vi "DrawFilledPolyOnImageGreyscale.vi"(4 "Thickness (Default: 1)":i32=1, 6 "Colour":u8=255, 7 "OpenCV Line Type (Default LINE_8)":T3=enum."LINE_8", 8 "error in (no error)":errorcluster, 9 "Point Type (Default: Any)":T1, 10 "Points":T2[](array[typedef]), 11 "Greyscale Image":refnum<data-value>) -> (0 "error out":errorcluster, 3 "Greyscale Image (Duplicate)":refnum<data-value>)   [LabVIEW 2020, in "g_ar_toolkit.image.lvlib"]
uses:
  g_ar_toolkit.image.lvlib
  Fill-Poly Points Type.ctl
  e24a04ad-8575-4d64-b8af-da4c51ecb9cd.vi
  Line Type.ctl
  g_ar_toolkit.common/Image Point (Integer).ctl
  g_ar_toolkit.common/g_ar_toolkit.common.lvlib
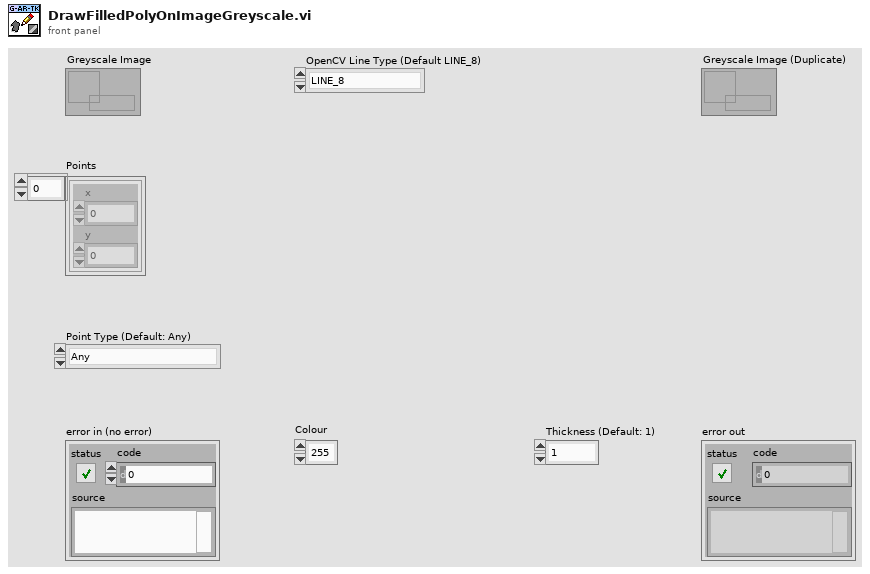
[diagram p1: front panel]
types:
  T1 = typedef "g_ar_toolkit.image.lvlib/Fill-Poly Points Type.ctl" = enum16{"Any", "Convex Only"}
  T2 = typedef "g_ar_toolkit.common.lvlib/Image Point (Integer).ctl" = cluster{"x":i32, "y":i32}
  T3 = typedef "g_ar_toolkit.image.lvlib/Line Type.ctl" = enum8{"FILLED", "LINE_4", "LINE_8", "LINE_AA"}
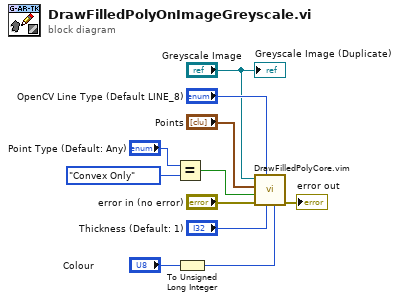
[diagram p0: block diagram]
diagram:
  n1 = Equal?(x="Point Type (Default: Any)", y=Fill-Poly_Points_Type."Convex Only") -> (x = y?=w2:bool)
  n2 = To Unsigned Long Integer(number="Colour") -> (unsigned 32bit integer=w6:u32)
  n3 = call "DrawFilledPolyCore.vim"("Colour"=w6, "Thickness"="Thickness (Default: 1)", "OpenCV Line Type"="OpenCV Line Type (Default LINE_8)", "error in (no error)"="error in (no error)", "Is Convex"=w2, "Points"="Points", "Src"="Greyscale Image") -> ("error out"=→"error out":errorcluster)  [unwired: 4 in]
  "Greyscale Image (Duplicate)" <- "Greyscale Image"
